vi "mav_connection_read.vi"(8 "error in":errorcluster, 9 "connection_type":enum16{"SERIAL", "TCP", "UDP"}(ring), 10 "bytes to read":u32, 11 "mav_connection_in":T2) -> (0 "error out":errorcluster, 2 "data out":string, 3 "mav_connection_out":T1)   [LabVIEW 2023]
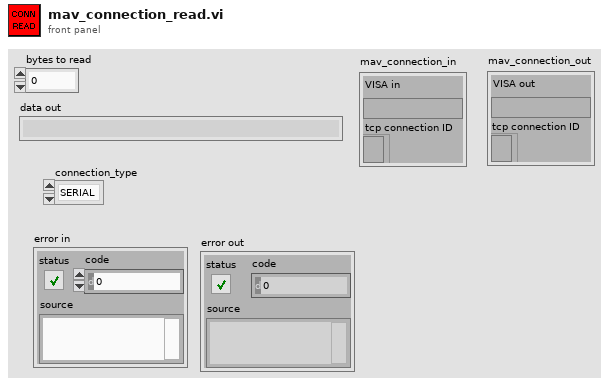
[diagram p1: front panel]
types:
  T1 = cluster{"VISA out":refnum<visa-resource-name>, "tcp connection ID":refnum<k5>}
  T2 = cluster{"VISA in":refnum<visa-resource-name>, "tcp connection ID":refnum<k5>}
  T3 = enum16{"Standard", "Buffered", "CRLF", "Immediate"}
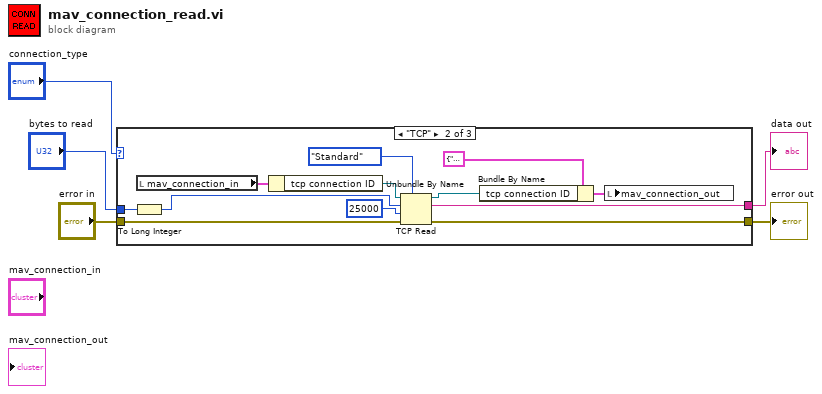
[diagram p0: block diagram]
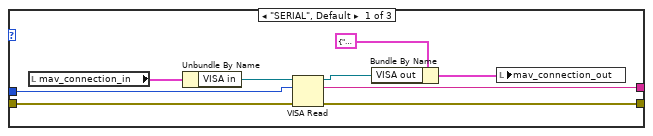
[diagram p2: hidden frame]
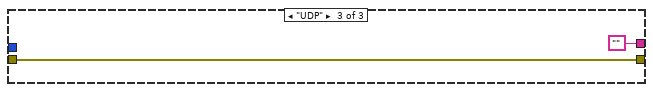
[diagram p3: hidden frame]
diagram:
  n1 = case shown="\"TCP\"" "connection_type" {
    tunnel: "error in" -> [w13 w22 w28]
    tunnel: [w14 w23 w28] -> w4
    tunnel: [w12 w24 ""] -> w2
    tunnel: "bytes to read" -> [w11 w21 _]
    frame "SERIAL", Default {
      n2 = local read "mav_connection_in"() -> (w10:T2)
      n3 = Unbundle By Name(w10) -> ("VISA in"=w9:refnum<visa-resource-name>)
      n4 = VISA Read(VISA resource name=w9, byte count=w11, error in (no error)=w13) -> (VISA resource name out=w6:refnum<visa-resource-name>, read buffer=w12:string, error out=w14:errorcluster)  [unwired: 1 out]
      n5 = Bundle By Name(cluster=T1 {"VISA out"="", "tcp connection ID"=refnum} ("mav_connection_out"), "VISA out"=w6) -> (w8:T1)
      n6 = local write "mav_connection_out"(w8) -> ()
    }
    frame "TCP" {
      n7 = To Long Integer(number=w21) -> (32bit integer=w20:i32)
      n8 = local read "mav_connection_in"() -> (w19:T2)
      n9 = Unbundle By Name(w19) -> ("tcp connection ID"=w18:refnum<k5>)
      n10 = TCP Read(connection ID=w18, bytes to read=w20, error in (no error)=w22, 7:T3."Standard" ("mode (standard)"), 9:25000 ("timeout ms (25000)")) -> (connection ID out=w15:refnum<k5>, data out=w24:string, error out=w23:errorcluster)
      n11 = Bundle By Name(cluster=T1 {"VISA out"="", "tcp connection ID"=refnum} ("mav_connection_out"), "tcp connection ID"=w15) -> (w17:T1)
      n12 = local write "mav_connection_out"(w17) -> ()
    }
    frame "UDP" {
    }
  }
  "error out" <- w4
  "data out" <- w2
